vi "READ.vi"(2 "Registers to Read":u8, 3 "Starting Address":u8 format="%02x", 4 "SPI Config In":T1) -> (0 "Frames Read":u8[](array[numeric]) format="%08b", 1 "SPI Config Out":T1)   [LabVIEW 2019]
uses:
  SPI/SPI Config.ctl
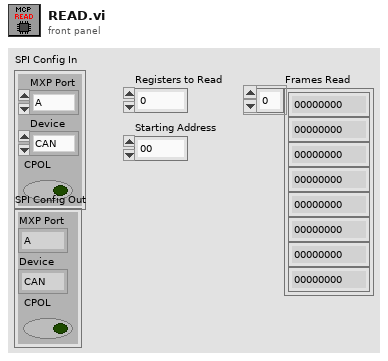
[diagram p1: front panel]
types:
  T1 = typedef "SPI Config.ctl" = cluster{"MXP Port":enum16{"A", "B"}, "Device":enum16{"CAN", "ENC", "IMU1", "IMU2"}, "CPOL":bool}
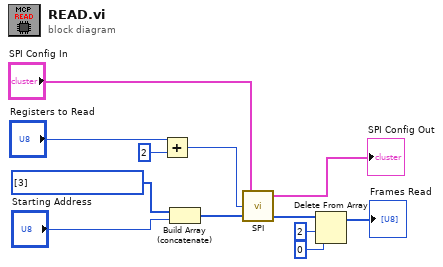
[diagram p0: block diagram]
diagram:
  n1 = Add(x="Registers to Read", y=u8 2) -> (x+y=w3:u8)
  n2 = Build Array (concatenate)(u8[] [3] ("Frames to Write"), "Starting Address") -> (w6:u8[])
  n3 = call "SPI.vi"("Data to Write"=w6, "Frames to Write"=w3, "SPI Config In"="SPI Config In") -> ("Data Read"=w1:u8[], "SPI Config Out"=→"SPI Config Out":T1)  [unwired: 1 out]
  n4 = Delete From Array(array=w1, length=2, index=0) -> (array with subset deleted=→"Frames Read":u8[])  [unwired: 1 out]
